vi "initialise.vi"(8 "error in (no error)":errorcluster, 11 "GenericPlugin in":refnum<class "SignalWriterDL101123SoundCard.lvclass">) -> (0 "error out":errorcluster, 3 "GenericPlugin out":refnum<class "SignalWriterDL101123SoundCard.lvclass">)   [LabVIEW 2010, in "SignalWriterDL101123SoundCard.lvclass"]
doc: "The dynamic dispatch-version of this VI initalises the plug-in object by allocating and initalising any dynamic resources need."
uses:
  SignalWriterDL101123SoundCard.lvclass
  GenericSignalWriter/GenericSignalWriter/GenericSignalWriter.lvclass
  SignalWriterDL101123SoundCard.lvclass/SignalWriterDL101123SoundCard.ctl
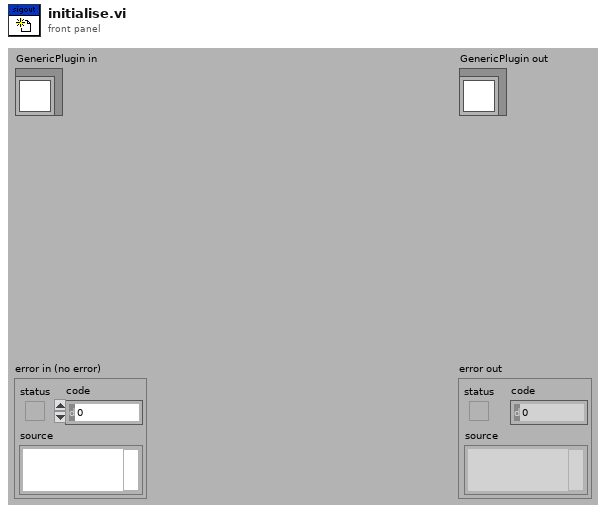
[diagram p1: front panel]
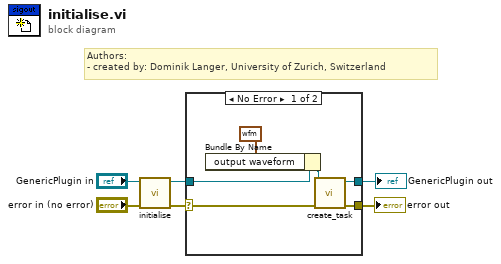
[diagram p0: block diagram]
diagram:
  # "Authors: \n- created by: Dominik Langer, University of Zurich, Switzerland"
  n1 = call-parent "initialise.vi"("error in (no error)"="error in (no error)", "GenericPlugin in"="GenericPlugin in") -> ("error out"=w1:errorcluster, "GenericPlugin out"=w2:refnum<class "SignalWriterDL101123SoundCard.lvclass">)  [unwired: 8 in]
  n2 = case shown="No Error" w1 {
    selector: w1 -> [w7 w14]
    tunnel: [w12 w14] -> w4
    tunnel: [w11 w13] -> w3
    tunnel: w2 -> [w10 w13]
    frame No Error {
      n3 = Bundle By Name(cluster=w10, "output waveform"=waveform(dbl) {"t0"=timestamp(0 s since 1904-01-01), "dt"=1.0, "Y"=[]}) -> (w9:refnum<class "SignalWriterDL101123SoundCard.lvclass">)
      n4 = call-dynamic "create_task.vi"("error in (no error)"=w7, "SignalWriterDL101123SoundCard in"=w9) -> ("error out"=w12:errorcluster, "SignalWriterDL101123SoundCard out"=w11:refnum<class "SignalWriterDL101123SoundCard.lvclass">)  [unwired: 8 in]
    }
    frame Error {
    }
  }
  "error out" <- w4
  "GenericPlugin out" <- w3
